vi "PointMap_Copy.vi"(8 "error in (no error)":errorcluster, 9 "Destination Map Name":string, 10 "Source Map Name":string) -> (0 "error out":errorcluster)   [LabVIEW 2017, in "PointValueMap.lvlib"]
doc: "Creates a copy of a point value map that includes the same point-value pairs as the original map."
uses:
  <vilib>/addons/PointValueMap/PointValueMap.lvlib
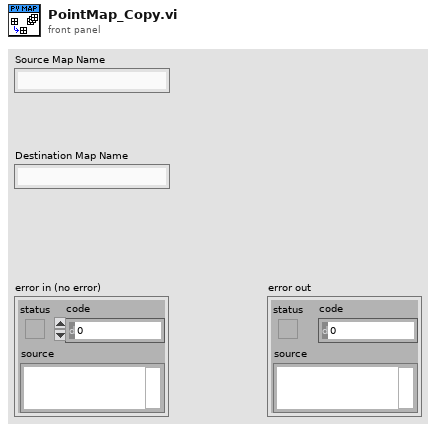
[diagram p1: front panel]
types:
  T1 = typedef "PointValueMap.lvlib/PointMap.ctl" = refnum<data-value>
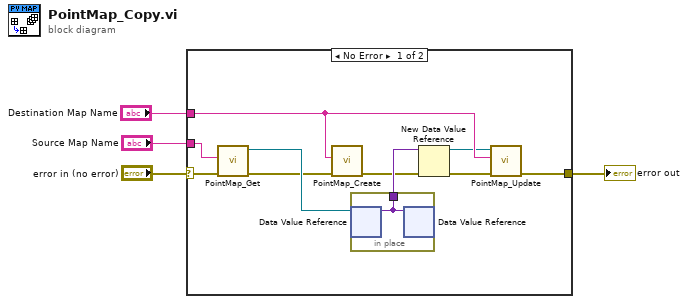
[diagram p0: block diagram]
diagram:
  n1 = case shown="No Error" "error in (no error)" {
    selector: "error in (no error)" -> [w9 w16]
    tunnel: "Source Map Name" -> [w14 _]
    tunnel: "Destination Map Name" -> [w12 _]
    tunnel: [w11 w16] -> w2
    frame No Error {
      n2 = call <vilib>:"PointMap_Get.vi"("error in (no error)"=w9, "Name"=w14) -> ("error out"=w10:errorcluster, "Map Out"=w13:T1)  [unwired: 7 in, 1 out]
      n3 = call <vilib>:"PointMap_Create.vi"("error in (no error)"=w10, "Name"=w12) -> ("error out"=w6:errorcluster)  [unwired: 8 in, 1 out]
      n4 = in-place {
        in-place-border: [w15] -> w8
        n5 = in-place-dvr #1(w13) -> (w15:variant)  [unwired: 1 out]
        n6 = in-place-dvr #1(w15) -> ()  [unwired: 2 out]
      }
      n7 = New Data Value Reference(data value=w8, error in=w6) -> (data value reference=w7:refnum<data-value>, error out=w5:errorcluster)
      n8 = call <vilib>:"PointMap_Update.vi"("error in (no error)"=w5, "Name"=w12, "Map"=w7) -> ("error out"=w11:errorcluster)  [unwired: 8 in]
    }
    frame Error {
    }
  }
  "error out" <- w2
